vi "rate safety.vi"(4 "Max Reverse Rate":dbl=50.0, 5 "Max Forward Rate":dbl=50.0, 6 "Desired Rate":dbl, 7 "Cutoff Rate":dbl=0.2, 8 "Encoder Rate":dbl) -> (0 "Encoder Error":bool, 1 "Excedded Rate Limit":bool, 2 "Output Rate":dbl, 3 "Encoder Rate Out":dbl)   [LabVIEW 2013]
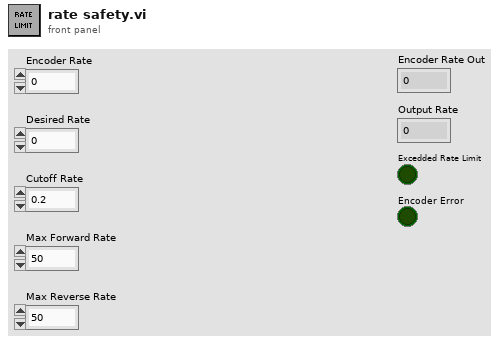
[diagram p1: front panel]
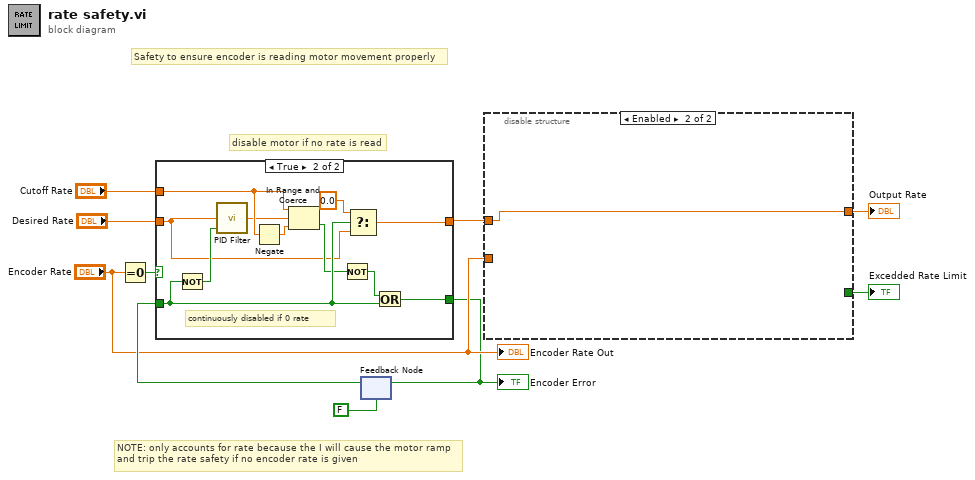
[diagram p0: block diagram]
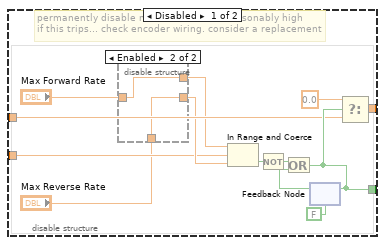
[diagram p2: hidden frame]
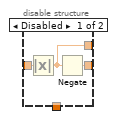
[diagram p3: hidden frame]
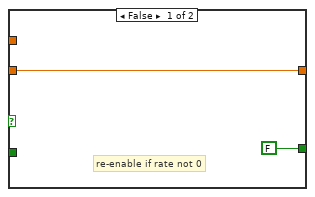
[diagram p4: hidden frame]
diagram:
  # "Safety to ensure encoder is reading motor movement properly"
  # "NOTE: only accounts for rate because the I will cause the motor ramp\nand trip the rate safety if no encoder rate is given"
  # "disable motor if no rate is read"
  n1 = Equal To 0?(x="Encoder Rate") -> (x = 0?=w9:bool)
  n2 = feedback #1(FALSE ("x > y?")) -> (w5:bool)
  n3 = case shown="True" w9 {
    tunnel: "Desired Rate" -> [w12 w13]
    tunnel: [w12 w22] -> w4
    tunnel: [FALSE w20] -> w1
    tunnel: w5 -> [_ w19]
    tunnel: "Cutoff Rate" -> [_ w17]
    frame False {
      # "re-enable if rate not 0"
    }
    frame True {
      # "continuously disabled if 0 rate"
      n4 = Not(x=w19) -> (.not. x?=w16:bool)
      n5 = call "PID Filter.vi"("reinitialize? (F)"=w16, "input"=w13) -> ("output"=w15:dbl)  [unwired: 3 in]
      n6 = Negate(x=w17) -> (-x=w18:dbl)
      n7 = In Range and Coerce(upper limit=w17, x=w15, lower limit=w18) -> (In Range?=w14:bool)  [unwired: 1 out]
      n8 = Not(x=w14) -> (.not. x?=w21:bool)
      n9 = Select(t=0.0, s=w19, f=w13) -> (s? t:f=w22:dbl)
      n10 = Or(x=w21, y=w19) -> (x .or. y?=w20:bool)
    }
  }
  "Encoder Error" <- w1
  n11 = feedback-in #1(w1) -> ()
  n12 = disable-structure shown="Enabled" {
    disable-tunnel: [w33 _] -> w8
    disable-tunnel: [w32 w42] -> w7
    disable-tunnel: w4 -> [w29 w42]
    disable-tunnel: "Encoder Rate" -> [w25 _]
    frame Disabled {
      # "permanently disable motor if rate is unreasonably high\nif this trips... check encoder wiring. consider a replacement"
      n13 = disable-structure shown="Enabled" {
        disable-tunnel: [w39 w41] -> w28
        disable-tunnel: "Max Forward Rate" -> [w38 w40]
        disable-tunnel: [w37 w40] -> w26
        disable-tunnel: "Max Reverse Rate" -> [_ w41]
        frame Disabled {
          n14 = Absolute Value(x=w38) -> (abs(x)=w37:dbl)
          n15 = Negate(x=w37) -> (-x=w39:dbl)
        }
        frame Enabled {
        }
      }
      n16 = In Range and Coerce(upper limit=w26, x=w25, lower limit=w28) -> (In Range?=w31:bool)  [unwired: 1 out]
      n17 = Not(x=w31) -> (.not. x?=w30:bool)
      n18 = feedback #2(FALSE ("x > y?")) -> (w34:bool)
      n19 = Or(x=w30, y=w34) -> (x .or. y?=w33:bool)
      n20 = feedback-in #2(w33) -> ()
      n21 = Select(t=0.0, s=w33, f=w29) -> (s? t:f=w32:dbl)
    }
    frame Enabled {
    }
  }
  "Output Rate" <- w7
  "Excedded Rate Limit" <- w8
  "Encoder Rate Out" <- "Encoder Rate"
